vi "demodulate_card.vi"(5 "Current/sensor index":i32 min=0 max=1 step=1, 6 "Raw data":dbl[][](array[numeric]), 7 "Reset":bool, 9 "Low carrier amplitudes":cdb[][](array[numeric]), 10 "Modulation info":T1 {"Hi channels at low" min=0 step=1; "Low carriers" format="%#_6p"; "High carriers" format="%#_6p"}, 11 "Config":T2={"IO params"={"Conversion"={"Rate"=0.0, "Num cards"=0, "Out channels"=0}, "Carriers"={"Phase shift"=0.0, "Levels"=[], "Delay samples"=0.0}, "TCP"={"Host"="192.168.1.15", "Port"=6666, "Buffering"=6, "Timeout"=6}, "Input channel sign"=[1, 1, 1]}, "High rate STFT"={"Win param"=0.0, "Window type"=0, "Win order"=0, "DFT size"=0, "Channels"=[], "Oversample"=0}, "Low rate STFT"={"Win param"=0.0, "Window type"=0, "Win order"=0, "DFT size"=0, "Channels"=[], "Oversample"=0}, "Filtering "=[]} {"Filtering"."Distortion"."Limit" format="%#_3p"; "Filtering"."Distortion"."LF cut" format="%#_3p"; "Filtering"."Kalman"."Measure noise" format="%#_3p"; "Filtering"."Kalman"."Process noise" format="%#_3p"; "Filtering"."Hum"."Limit" format="%#_3p"; "Filtering"."Hum"."Frequency" format="%#_4p"; "Low rate STFT"."Oversample" min=1 step=1; "Low rate STFT"."Channels" min=0 step=1; "Low rate STFT"."DFT size" min=1 step=1; "Low rate STFT"."Window type" items=["Rectangle"=0, "Hanning"=1, "Hamming"=2, "Blackman-Harris"=3, "Exact Blackman"=4, "Blackman"=5, "Flat Top"=6, "4 Term B-Harris "=7, "7 Term B-Harris"=8, "Low Sidelobe"=9, "Blackman Nuttall"=11, "Triangle"=30, "Bartlett-Hanning"=31, "Bohman"=32, "Parzen"=33, "Welch"=34, "Kaiser"=60, "Dolph-Chebyshev"=61, "Gaussian"=62]; "High rate STFT"."Oversample" min=1 step=1; "High rate STFT"."Channels" min=0 step=1; "High rate STFT"."DFT size" min=1 step=1; "High rate STFT"."Window type" items=["Rectangle"=0, "Hanning"=1, "Hamming"=2, "Blackman-Harris"=3, "Exact Blackman"=4, "Blackman"=5, "Flat Top"=6, "4 Term B-Harris "=7, "7 Term B-Harris"=8, "Low Sidelobe"=9, "Blackman Nuttall"=11, "Triangle"=30, "Bartlett-Hanning"=31, "Bohman"=32, "Parzen"=33, "Welch"=34, "Kaiser"=60, "Dolph-Chebyshev"=61, "Gaussian"=62]; "IO params"."Input channel sign" min=-1 max=1 step=1; "IO params"."Carriers"."Levels" min=0.0 step=0.1; "IO params"."Conversion"."Rate" format="%#_8g"}) -> (2 "High carrier amplitudes":cdb[][][](array[numeric]), 3 "Trace channels":T8[](array[typedef]))   [LabVIEW 2026]
uses:
  gui/trace_channel.ctl
  ilemt_config.ctl
  system/IO_params.ctl
  stft_params.ctl
  <vilib>/Analysis/4window.llb/windowTd.ctl
  filter_params.ctl
  detrend_mode.ctl
  modulation_info.ctl
  <vilib>/Analysis/NI_AALPro.lvlib
panel:
  # "Sample"
  # "High (Fd) rate carrier amplitudes for one card."
  # "Carrier"
  # "Channel"
  # "Carrier"
  # "Coupling matrix for the previous low carrier amplitudes."
  # "Channel"
  # "Channel"
  # "Full  (Fs) rate input data"
  # "Sample"
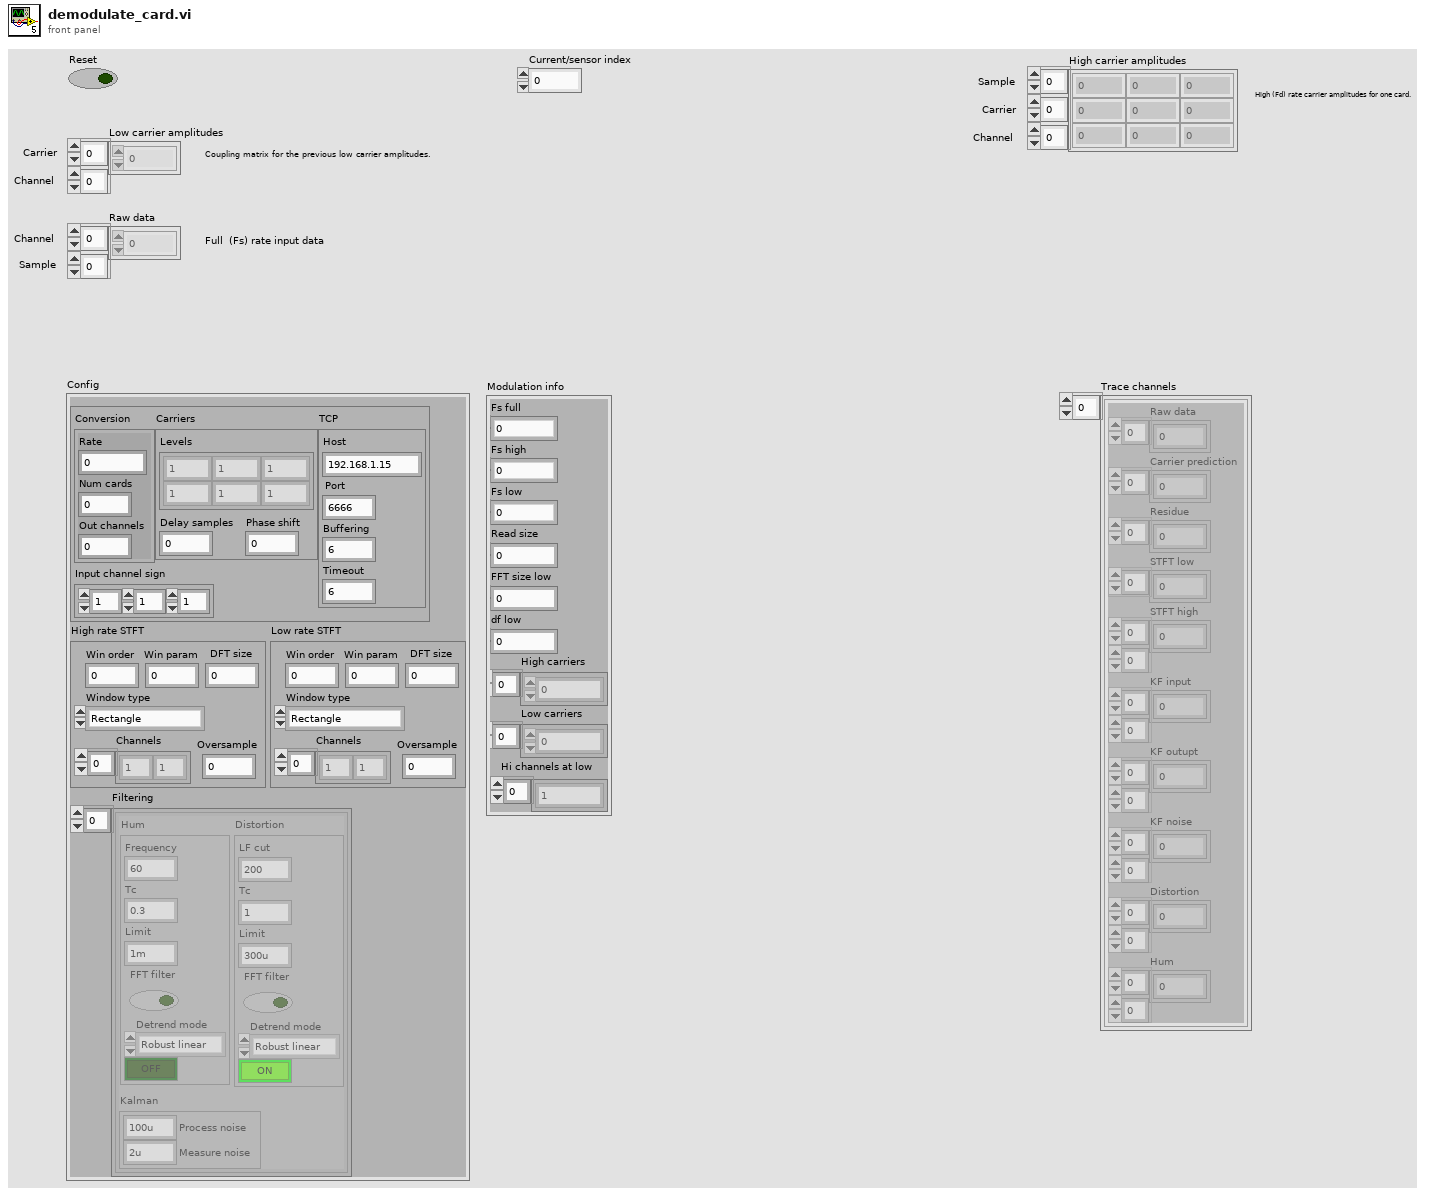
[diagram p1: front panel]
types:
  T1 = typedef "modulation_info.ctl" = cluster{"Fs full":dbl, "Fs high":dbl, "Fs low":dbl, "Read size":i32, "FFT size low":i32, "df low":dbl, "High carriers":dbl[], "Low carriers":dbl[], "Hi channels at low":i32[]}
  T2 = typedef "ilemt_config.ctl" = cluster{"IO params":T3, "High rate STFT":T4, "Low rate STFT":T4, "Filtering ":T6[]}
  T3 = typedef "IO_params.ctl" = cluster{"Conversion":cluster{"Rate":dbl, "Num cards":u32, "Out channels":u32}, "Carriers":cluster{"Phase shift":dbl, "Levels":dbl[][], "Delay samples":dbl}, "TCP":cluster{"Host":string, "Port":i32, "Buffering":u32, "Timeout":u32}, "Input channel sign":i32[]}
  T4 = typedef "stft_params.ctl" = cluster{"Win param":dbl, "Window type":T5, "Win order":i32, "DFT size":i32, "Channels":i32[], "Oversample":i32}
  T5 = typedef "NI_AALPro.lvlib/windowTd.ctl" = u32
  T6 = typedef "filter_params.ctl" = cluster{"Hum":cluster{"Frequency":dbl, "Tc":dbl, "Limit":dbl, "FFT filter":bool, "Detrend mode":T7, "Enable":bool}, "Kalman":cluster{"Process noise":dbl, "Measure noise":dbl}, "Distortion":cluster{"LF cut":dbl, "Tc":dbl, "Limit":dbl, "FFT filter":bool, "Detrend mode":T7, "Enable":bool}}
  T7 = typedef "detrend_mode.ctl" = enum16{"Zero mean", "Linear", "Robust linear"}
  T8 = typedef "trace_channel.ctl" = cluster{"Raw data":dbl[], "Carrier prediction":dbl[], "Residue":dbl[], "STFT low":cdb[], "STFT high":cdb[][], "KF input":cdb[][], "KF outupt":cdb[][], "KF noise":dbl[][], "Distortion":cdb[][], "Hum":cdb[][]}
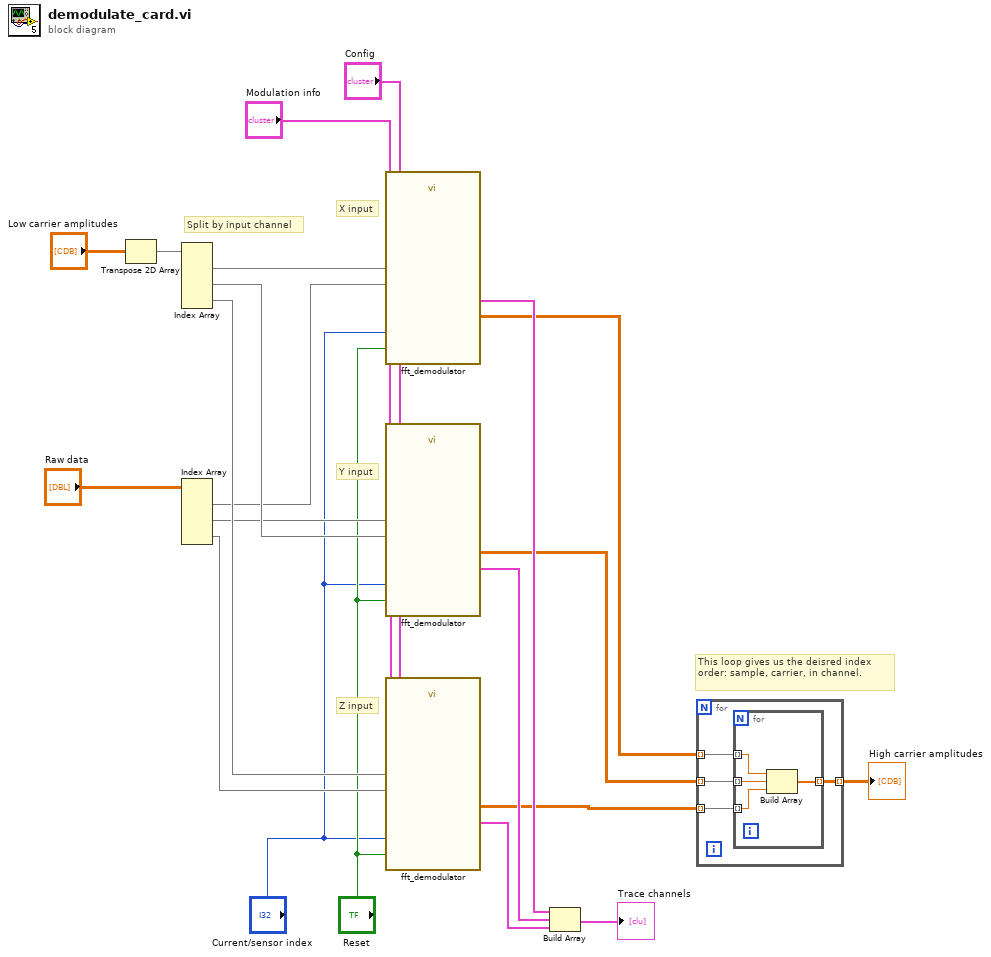
[diagram p0: block diagram]
diagram:
  # "This loop gives us the deisred index order: sample, carrier, in channel."
  # "Z input"
  # "Y input"
  # "X input"
  # "Split by input channel"
  n1 = Transpose 2D Array(2D array="Low carrier amplitudes") -> (transposed array=w6:cdb[][])
  n2 = Index Array(array=w6) -> (element #1=w10:cdb[], element #2=w14:cdb[], element #3=w15:cdb[])  [unwired: 6 in]
  n3 = Index Array(array="Raw data") -> (element #1=w11:dbl[], element #2=w12:dbl[], element #3=w13:dbl[])  [unwired: 6 in]
  n4 = call "fft_demodulator.vi"("Reset"="Reset", "Config"="Config", "Modulation info"="Modulation info", "Low carrier amplitudes"=w10, "Raw data"=w11, "Current/sensor index"="Current/sensor index") -> ("High carrier amplitudes"=w5:cdb[][], "Trace channel out"=w16:T8)  [unwired: 8 in]
  n5 = call "fft_demodulator.vi"("Reset"="Reset", "Config"="Config", "Modulation info"="Modulation info", "Low carrier amplitudes"=w14, "Raw data"=w12, "Current/sensor index"="Current/sensor index") -> ("High carrier amplitudes"=w4:cdb[][], "Trace channel out"=w17:T8)  [unwired: 8 in]
  n6 = call "fft_demodulator.vi"("Reset"="Reset", "Config"="Config", "Modulation info"="Modulation info", "Low carrier amplitudes"=w15, "Raw data"=w13, "Current/sensor index"="Current/sensor index") -> ("High carrier amplitudes"=w3:cdb[][], "Trace channel out"=w18:T8)  [unwired: 8 in]
  n7 = Build Array(w16, w17, w18) -> (→"Trace channels":T8[])
  n8 = for {
    tunnel: w5 -> [w23] mode=indexing
    tunnel: w4 -> [w24] mode=indexing
    tunnel: w3 -> [w25] mode=indexing
    tunnel: [w22] -> w2 mode=indexing
    n9 = for {
      tunnel: w25 -> [w28] mode=indexing
      tunnel: w24 -> [w29] mode=indexing
      tunnel: w23 -> [w27] mode=indexing
      tunnel: [w26] -> w22 mode=indexing
      n10 = Build Array(w27, w29, w28) -> (w26:cdb[])
    }
  }
  "High carrier amplitudes" <- w2
